vi "Teleop.vi"(10 "Match Info":T1={"Autonomous Elapsed Seconds"=0.0, "TeleOp Elapsed Seconds"=0.0, "Disabled Elapsed Seconds"=0.0, "Visited Autonomous"=FALSE, "Visited TeleOp"=FALSE, "Visited Disabled"=FALSE, "Autonomous Settings"={"Autonomous Style"=enum."Independent", "VI Refnum"=refnum}}, 11 "Call Context":T2) -> ()   [LabVIEW 2019]
doc: "This VI is called for each TeleOp packet received from the DS where the robot is not disabled. It is often used to read from the joysticks and update I/O or to update setpoints for timed control loops. It should complete and return within 20 milliseconds or it may miss DS packets."
uses:
  <vilib>/Rock Robotics/WPI/DriverStation/WPI_DriverStationDerivedRobotMode.ctl
  <vilib>/Rock Robotics/WPI/DriverStation/WPI_DriverStationMatch Info.ctl
  <vilib>/Rock Robotics/WPI/Solenoid/WPI_SolenoidValue.ctl
  <vilib>/Rock Robotics/WPI/ThirdParty/Phoenix-LabVIEW/Motor Controller/Controls/CTRE_Phoenix_MotorControl_ControlMode.ctl
  <vilib>/Rock Robotics/WPI/Utilities/WPI_GetSetVariantRefNum.vi
  <vilib>/Rock Robotics/Network Tables/NT Write Boolean Array.vi
  <vilib>/Rock Robotics/Network Tables/NT Write Numeric Array.vi
  <vilib>/Rock Robotics/Network Tables/NT Read Boolean.vi
  <vilib>/Rock Robotics/Network Tables/NT Read Number.vi
  <vilib>/Rock Robotics/WPI/Solenoid/WPI_SolenoidSetEnum.vi
  <vilib>/addons/control/pid/pid.llb/PID (DBL).vi
  <vilib>/Rock Robotics/Network Tables/NT Write Number.vi
  <vilib>/addons/control/pid/NI_PID_pid.lvlib
panel:
  out "Sample Slider 0":dbl(slide) scale=0.0..5.0
  out "Sample Boolean 1":bool
  out "Sample Boolean 0":bool
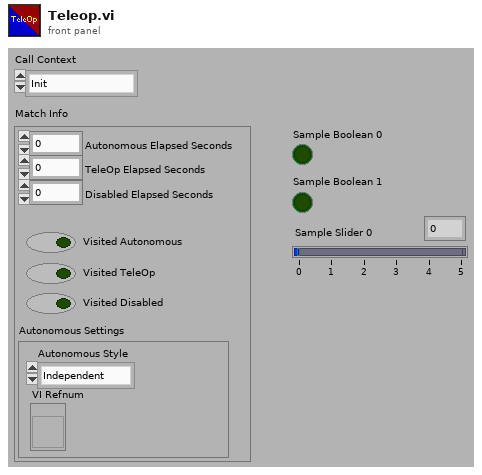
[diagram p1: front panel]
types:
  T1 = typedef "WPI_DriverStationMatch Info.ctl" = cluster{"Autonomous Elapsed Seconds":dbl, "TeleOp Elapsed Seconds":dbl, "Disabled Elapsed Seconds":dbl, "Visited Autonomous":bool, "Visited TeleOp":bool, "Visited Disabled":bool, "Autonomous Settings":cluster{"Autonomous Style":enum16{"Iterative", "Independent"}, "VI Refnum":refnum<vi>}}
  T2 = typedef "WPI_DriverStationDerivedRobotMode.ctl" = enum16{"Init", "Execute", "Stop"}
  T3 = typedef "CTRE_Phoenix_MotorControl_ControlMode.ctl" = u16
  T4 = typedef "WPI_SolenoidValue.ctl" = enum16{"Off", "On", "Forward", "Reverse"}
  T5 = typedef "WPI_RobotDriveDevRef.ctl" = cluster{"DevStatus":errorcluster, "Motors[]":T6[], "Square Inputs":bool, "Max Output":dbl}
  T6 = typedef "WPI_MotorControlDeviceRef.ctl" = cluster{"DeviceStatus":errorcluster, "Type":T7, "PWM":cluster{"PWM Channel":T8, "DeadBand":T9}, "CAN":cluster{"Device Number":u8, "SetOutput VI Ref":variant, "GetOutput VI Ref":variant, "Enable VI Ref":variant, "Disable VI Ref":variant, "Data":variant}, "Invert":bool, "DIO PWM":cluster{"PWM \"Enable\" Channel":T8, "DIOChannel":T10, "PWM Rate":dbl}}
  T7 = typedef "WPI_MotorControlType.ctl" = enum16{"PWM", "CAN", "DIO PWM"}
  T8 = typedef "FPGA_DIOPWMChannel.ctl" = enum8{"PWM 0", "PWM 1", "PWM 2", "PWM 3", "PWM 4", "PWM 5", "PWM 6", "PWM 7", "PWM 8", "PWM 9", "PWM MXP 0", "PWM MXP 1", "PWM MXP 2", "PWM MXP 3", "PWM MXP 4", "PWM MXP 5", "PWM MXP 6", "PWM MXP 7", "PWM MXP 8", "PWM MXP 9", "Invalid"}
  T9 = typedef "WPI_PWMDeadband.ctl" = cluster{"Name":string, "maxPositivePwm":i32, "minPositivePwm":i32, "centerPwm":i32, "maxNegativePwm":i32, "minNegativePwm":i32, "angularRange":u16}
  T10 = typedef "FPGA_DIOChannel.ctl" = enum8{"DIO 0", "DIO 1", "DIO 2", "DIO 3", "DIO 4", "DIO 5", "DIO 6", "DIO 7", "DIO 8", "DIO 9", "DIO MXP 0", "DIO MXP 1", "DIO MXP 2", "DIO MXP 3", "DIO MXP 4", "DIO MXP 5", "DIO MXP 6", "DIO MXP 7", "DIO MXP 8", "DIO MXP 9", "DIO MXP 10", "DIO MXP 11", "DIO MXP 12", "DIO MXP 13", "DIO MXP 14", "DIO MXP 15", "SPI Port CS1", "SPI Port CS2", "SPI Port CS3", "SPI Port MISO", "SPI Port MOSI", "Invalid"}
  T11 = typedef "WPI_JoystickDevRef.ctl" = cluster{"Device":T12}
  T12 = typedef "WPI_JoystickDeviceEnum.ctl" = enum16{"USB 0", "USB 1", "USB 2", "USB 3", "USB 4", "USB 5"}
  T13 = cluster{"Buttons[0]":bool, "Buttons[1]":bool, "Buttons[2]":bool, "Buttons[3]":bool, "Buttons[4]":bool, "Buttons[5]":bool, "Buttons[6]":bool, "Buttons[7]":bool, "Buttons[8]":bool}
  T14 = typedef "WPI_SolenoidDevRef.ctl" = cluster{"DevStatus":errorcluster, "Pneumatics Control Module":u8, "Forward Solenoid Channel":T15, "Reverse Solenoid Channel":T15}
  T15 = typedef "WPI_SolenoidChannel.ctl" = enum8{"Solenoid 0", "Solenoid 1", "Solenoid 2", "Solenoid 3", "Solenoid 4", "Solenoid 5", "Solenoid 6", "Solenoid 7", "Invalid"}
  T16 = cluster{"proportional gain (Kc)":dbl, "integral time (Ti, min)":dbl, "derivative time (Td, min)":dbl}
  T17 = typedef "WPI_SwitchDevRef.ctl" = cluster{"DevStatus":errorcluster, "DIO Channel":T10, "CntIndex":T18, "Normally Closed":bool}
  T18 = typedef "FPGA_CounterCtrSystemIndex.ctl" = enum8{"Ctr 0", "Ctr 1", "Ctr 2", "Ctr 3", "Ctr 4", "Ctr 5", "Ctr 6", "Ctr 7", "Invalid"}
  T19 = typedef "WPI_DigitalInputDevRef.ctl" = cluster{"DevStatus":errorcluster, "DIO Channel":T10}
  T20 = typedef "WPI_EncoderDevRef.ctl" = cluster{"DevStatus":errorcluster, "EncoderIndex":T21, "CounterIndex":T18, "DistancePerCount":dbl, "Decoding Type":T22}
  T21 = typedef "FPGA_EncoderIdx.ctl" = enum8{"Enc 0", "Enc 1", "Enc 2", "Enc 3", "Enc 4", "Enc 5", "Enc 6", "Enc 7", "Invalid"}
  T22 = typedef "WPI_EncoderType.ctl" = enum16{"1x", "2x", "4x"}
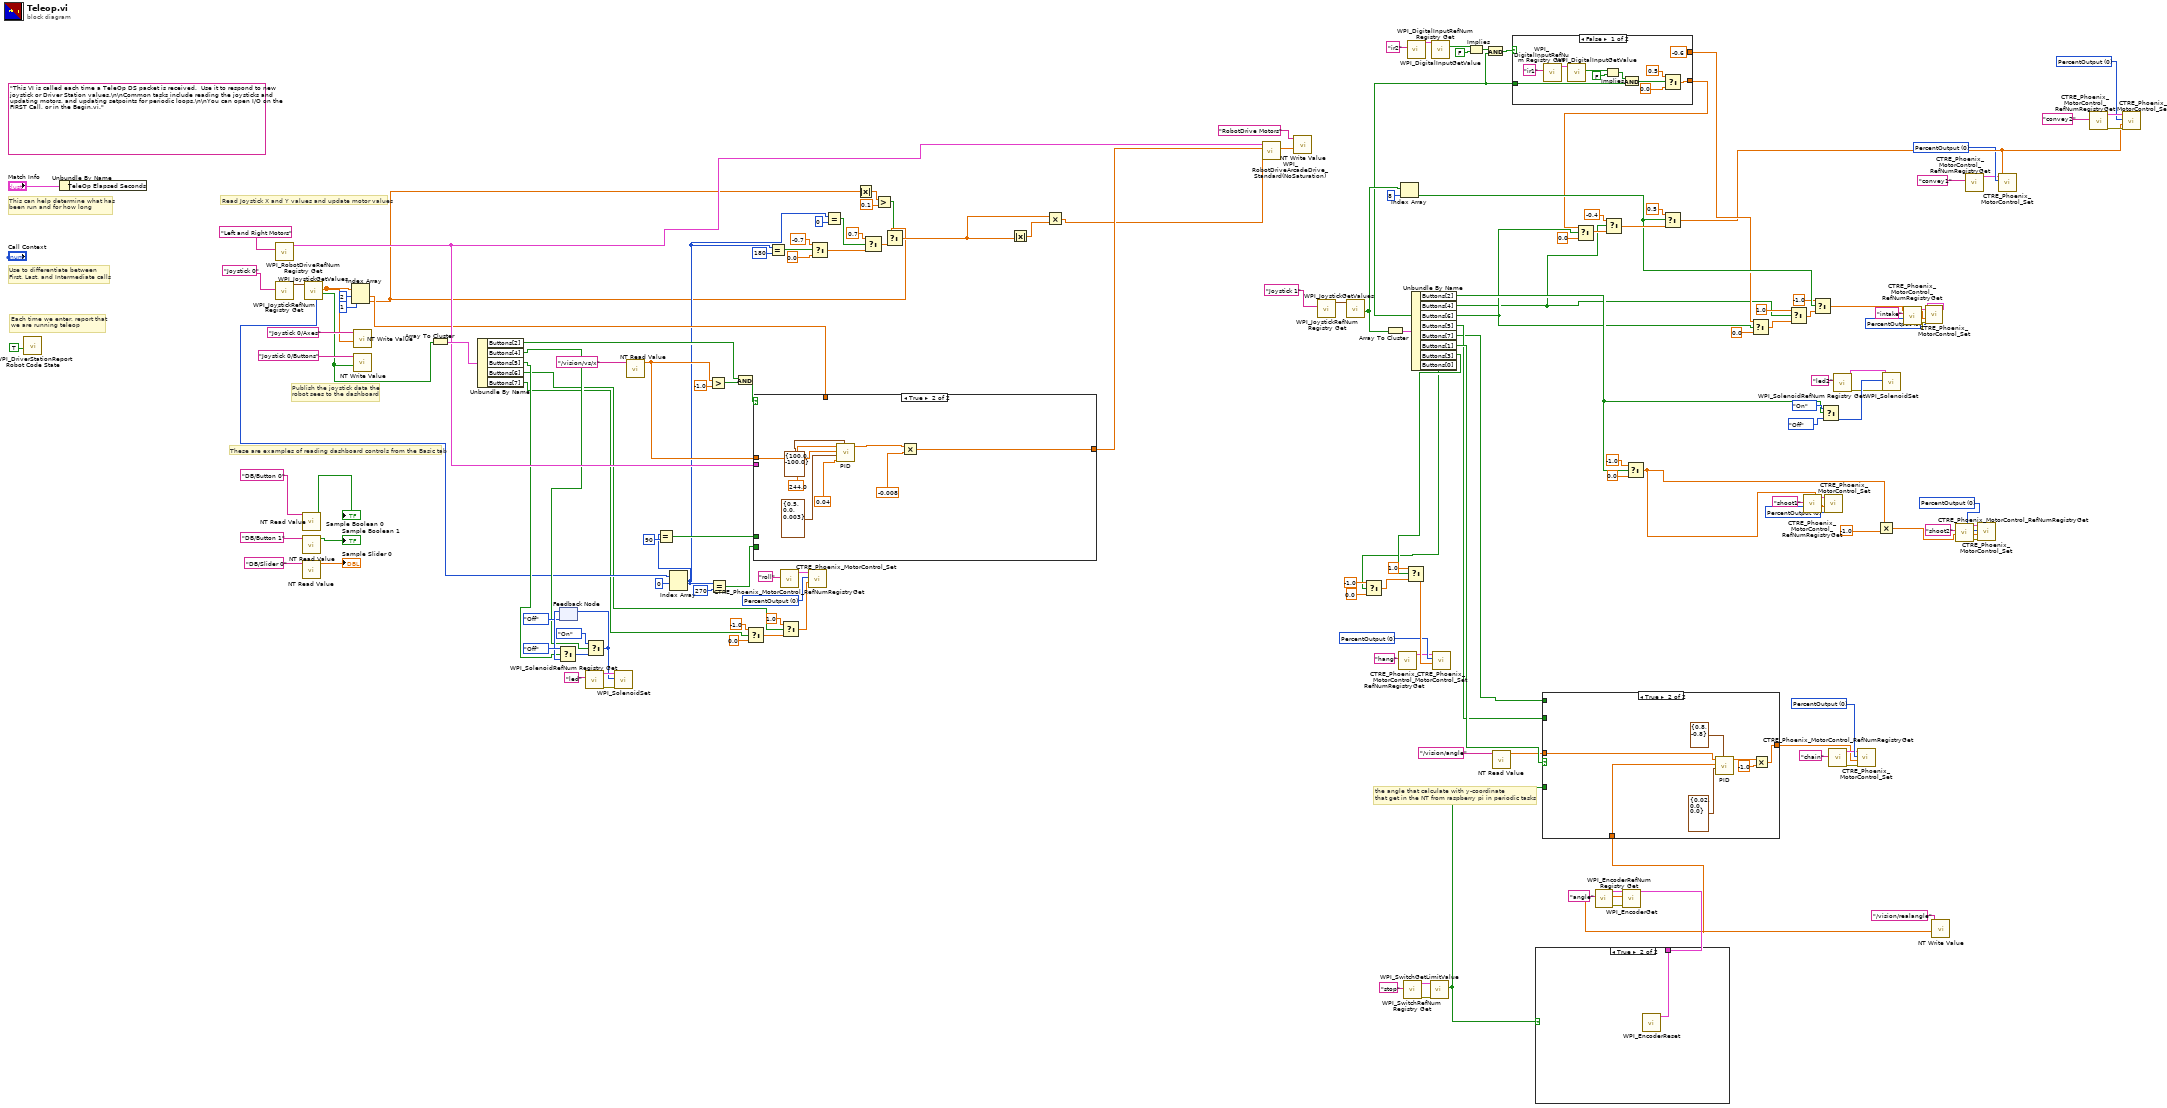
[diagram p0: block diagram]
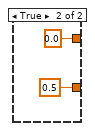
[diagram p2: hidden frame]
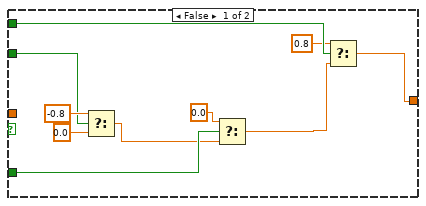
[diagram p3: hidden frame]
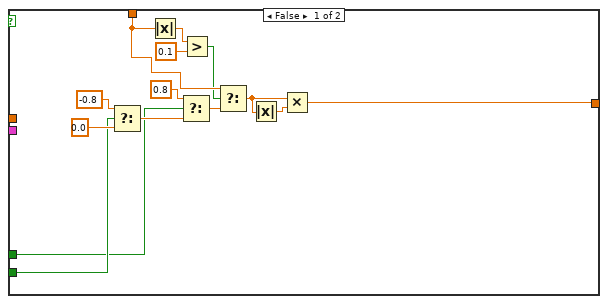
[diagram p5: hidden frame]
diagram:
  w4 = T3 0 items=["PercentOutput"=0, "Position"=1, "Velocity"=2, "Current"=3, "Follower"=5, "MotionProfile"=6, "MotionMagic"=7, "MotionProfileArc"=10, "Disabled"=15] ("Control Mode")
  w7 = T3 0 items=["PercentOutput"=0, "Position"=1, "Velocity"=2, "Current"=3, "Follower"=5, "MotionProfile"=6, "MotionMagic"=7, "MotionProfileArc"=10, "Disabled"=15] ("Control Mode")
  w34 = T3 0 items=["PercentOutput"=0, "Position"=1, "Velocity"=2, "Current"=3, "Follower"=5, "MotionProfile"=6, "MotionMagic"=7, "MotionProfileArc"=10, "Disabled"=15] ("Control Mode")
  w39 = T3 0 items=["PercentOutput"=0, "Position"=1, "Velocity"=2, "Current"=3, "Follower"=5, "MotionProfile"=6, "MotionMagic"=7, "MotionProfileArc"=10, "Disabled"=15] ("Control Mode")
  w85 = T3 0 items=["PercentOutput"=0, "Position"=1, "Velocity"=2, "Current"=3, "Follower"=5, "MotionProfile"=6, "MotionMagic"=7, "MotionProfileArc"=10, "Disabled"=15] ("Control Mode")
  w102 = T3 0 items=["PercentOutput"=0, "Position"=1, "Velocity"=2, "Current"=3, "Follower"=5, "MotionProfile"=6, "MotionMagic"=7, "MotionProfileArc"=10, "Disabled"=15] ("Control Mode")
  w114 = T3 0 items=["PercentOutput"=0, "Position"=1, "Velocity"=2, "Current"=3, "Follower"=5, "MotionProfile"=6, "MotionMagic"=7, "MotionProfileArc"=10, "Disabled"=15] ("Control Mode")
  w132 = T3 0 items=["PercentOutput"=0, "Position"=1, "Velocity"=2, "Current"=3, "Follower"=5, "MotionProfile"=6, "MotionMagic"=7, "MotionProfileArc"=10, "Disabled"=15] ("Control Mode")
  (unwired) "This VI is called each time a TeleOp DS packet is received.  Use it to respond to new joystick or Driver Station values.\n\nCommon tasks include reading the joysticks and updating motors, and updating setpoints for periodic loops.\n\nYou can open I/O on the FIRST Call, or in the Begin.vi."
  # "the angle that calculate with y-coordinate\nthat get in the NT from raspberry pi in periodic tasks"
  # "These are examples of reading dashboard controls from the Basic tab"
  # "Publish the joystick data the\nrobot sees to the dashboard"
  # "Each time we enter, report that\nwe are running teleop"
  # "Use to differentiate between\nFirst, Last, and Intermediate calls"
  # "This can help determine what has\nbeen run and for how long"
  # "Read Joystick X and Y values and update motor values"
  n1 = call <vilib>:"WPI_DriverStationReport Robot Code State.vi"("TeleOp"=TRUE ("Autonomous")) -> ()  [unwired: 10 in, 1 out]
  n2 = Unbundle By Name("Match Info") -> ()  [unwired: 1 out]
  n3 = call <vilib>:"WPI_RobotDriveRefNum Registry Get.vi"("refnum name"="Left and Right Motors") -> ("RobotDriveDevRef"=w143:T5)  [unwired: 1 in, 9 out]
  n4 = call <vilib>:"WPI_JoystickRefNum Registry Get.vi"("refnum name"="Joystick 0") -> ("JoystickDevRef"=w158:T11)  [unwired: 1 in, 9 out]
  n5 = call-poly <vilib>:"NT Read Value.vi"("Name"="DB/Button 0" ("refnum name")) -> ("Boolean"=→"Sample Boolean 0":bool)  [unwired: 9 in, 1 out]
  n6 = call-poly <vilib>:"NT Read Value.vi"("Name"="DB/Slider 0" ("refnum name")) -> ("Numeric"=→"Sample Slider 0":dbl)  [unwired: 9 in, 1 out]
  n7 = call-poly <vilib>:"NT Read Value.vi"("Name"="DB/Button 1" ("refnum name")) -> ("Boolean"=→"Sample Boolean 1":bool)  [unwired: 9 in, 1 out]
  n8 = call <vilib>:"WPI_JoystickGetValues.vi"("JoystickDevRef"=w158) -> ("Buttons"=w145:bool[], "Axes"=w154:dbl[], "POVs"=w79:i16[])  [unwired: 6 in, 2 out]
  n9 = Index Array(array=w154, index #1=2 ("index"), index #2=1 ("index")) -> (element #1=w94:dbl, element #2=w57:dbl)
  n10 = call-poly <vilib>:"NT Write Value.vi"("Numeric Array"=w154, "Name"="Joystick 0/Axes") -> ()  [unwired: 9 in, 1 out]
  n11 = call-poly <vilib>:"NT Write Value.vi"("Boolean Array"=w145, "Name"="Joystick 0/Buttons") -> ()  [unwired: 9 in, 1 out]
  n12 = Array To Cluster(array=w145) -> (cluster=w144:T13)
  n13 = Unbundle By Name(w144) -> ("Buttons[2]"=w96:bool, "Buttons[4]"=w116:bool, "Buttons[5]"=w115:bool, "Buttons[6]"=w72:bool, "Buttons[7]"=w71:bool)
  n14 = feedback #1(WPI_SolenoidValue."Off" ("Value")) -> (w119:T4)
  n15 = Select(t=WPI_SolenoidValue."Off" ("Value"), s=w115, f=w119) -> (s? t:f=w120:T4)
  n16 = call <vilib>:"WPI_SolenoidRefNum Registry Get.vi"("refnum name"="led") -> ("error out"=w125:errorcluster, "SolenoidDevRef"=w124:T14)  [unwired: 9 in]
  n17 = Select(t=WPI_SolenoidValue."On" ("Value"), s=w116, f=w120) -> (s? t:f=w117:T4)
  n18 = feedback-in #1(w117) -> ()
  n19 = call-poly <vilib>:"WPI_SolenoidSet.vi"("error in (no error)"=w125, "Value"=w117, "SolenoidDevRef"=w124) -> ()  [unwired: 7 in, 2 out]
  n20 = call-poly <vilib>:"NT Read Value.vi"("Name"="/vision/vs/x") -> ("Numeric"=w99:dbl)  [unwired: 9 in, 1 out]
  n21 = Index Array(array=w79, index #1=0 ("index")) -> (element #1=w61:i16)  [unwired: 1 in, 1 out]
  n22 = Equal?(x=w61, y=i16 90) -> (x = y?=w76:bool)
  n23 = Greater?(x=w99, y=-1.0) -> (0:w97:bool)
  n24 = Equal?(x=w61, y=i16 270) -> (x = y?=w77:bool)
  n25 = And(x=w96, y=w97) -> (x .and. y?=w95:bool)
  n26 = Select(t=-1.0, s=w71, f=0.0) -> (s? t:f=w82:dbl)
  n27 = case shown="True" w95 {
    tunnel: w143 -> [_ _]
    tunnel: w99 -> [_ w183]
    tunnel: [w162 w177] -> w93
    tunnel: w94 -> [w166 _]
    tunnel: w77 -> [w170 _]
    tunnel: w76 -> [w169 _]
    frame False {
      n28 = Select(t=-0.8, s=w170, f=0.0) -> (s? t:f=w174:dbl)
      n29 = Absolute Value(x=w166) -> (abs(x)=w165:dbl)
      n30 = Select(t=0.8, s=w169, f=w174) -> (s? t:f=w171:dbl)
      n31 = Greater?(x=w165, y=0.1) -> (0:w163:bool)
      n32 = Select(t=w166, s=w163, f=w171) -> (s? t:f=w167:dbl)
      n33 = Absolute Value(x=w167) -> (abs(x)=w168:dbl)
      n34 = Multiply(x=w167, y=w168) -> (x*y=w162:dbl)
    }
    frame True {
      n35 = call-poly <vilib>:"PID.vi"("output range"=cluster{"output high":dbl, "output low":dbl} {"output high"=100.0, "output low"=-100.0}, "dt (s)"=0.04, "PID gains"=T16 {"proportional gain (Kc)"=0.5, "integral time (Ti, min)"=0.0, "derivative time (Td, min)"=0.003}, "process variable"=w183, "setpoint"=244.0) -> ("output"=w179:dbl)  [unwired: 5 in, 1 out]
      n36 = Multiply(x=w179, y=-0.008) -> (x*y=w177:dbl)
    }
  }
  n37 = Equal?(x=w61, y=i16 180) -> (x = y?=w62:bool)
  n38 = call <vilib>:"CTRE_Phoenix_MotorControl_RefNumRegistryGet.vi"("refnum name"="roll") -> ("PhoenixMotorControlDevRef"=w87:T6)  [unwired: 9 in, 1 out]
  n39 = Select(t=1.0, s=w72, f=w82) -> (s? t:f=w78:dbl)
  n40 = call <vilib>:"CTRE_Phoenix_MotorControl_Set.vi"("Output"=w78, "Control Mode"=w85, "PhoenixMotorControlDevRef"=w87) -> ()  [unwired: 7 in, 2 out]
  n41 = Select(t=-0.7, s=w62, f=0.0) -> (s? t:f=w67:dbl)
  n42 = Equal?(x=w61, y=i16 0) -> (x = y?=w63:bool)
  n43 = Absolute Value(x=w57) -> (abs(x)=w56:dbl)
  n44 = Select(t=0.7, s=w63, f=w67) -> (s? t:f=w70:dbl)
  n45 = Greater?(x=w56, y=0.1) -> (0:w54:bool)
  n46 = Select(t=w57, s=w54, f=w70) -> (s? t:f=w59:dbl)
  n47 = Absolute Value(x=w59) -> (abs(x)=w60:dbl)
  n48 = Multiply(x=w59, y=w60) -> (x*y=w58:dbl)
  n49 = call <vilib>:"WPI_RobotDriveArcadeDrive_Standard(NoSaturation).vi"("Y axis value"=w58, "X axis value"=w93, "RobotDriveDevRef"=w143) -> ("Motor Values"=w147:dbl[])  [unwired: 1 in, 7 out]
  n50 = call-poly <vilib>:"NT Write Value.vi"("Numeric Array"=w147, "Name"="RobotDrive Motors") -> ()  [unwired: 9 in, 1 out]
  n51 = call <vilib>:"WPI_JoystickRefNum Registry Get.vi"("refnum name"="Joystick 1") -> ("JoystickDevRef"=w139:T11)  [unwired: 1 in, 9 out]
  n52 = call <vilib>:"WPI_JoystickGetValues.vi"("JoystickDevRef"=w139) -> ("Buttons"=w47:bool[])  [unwired: 6 in, 4 out]
  n53 = Array To Cluster(array=w47) -> (cluster=w137:T13)
  n54 = call <vilib>:"CTRE_Phoenix_MotorControl_RefNumRegistryGet.vi"("refnum name"="hang") -> ("PhoenixMotorControlDevRef"=w100:T6)  [unwired: 9 in, 1 out]
  n55 = Index Array(array=w47, index=8) -> (element=w44:bool)
  n56 = call <vilib>:"WPI_SwitchRefNum Registry Get.vi"("refnum name"="stop") -> ("error out"=w90:errorcluster, "SwitchDevRef"=w89:T17)  [unwired: 9 in]
  n57 = call <vilib>:"WPI_DigitalInputRefNum Registry Get.vi"("refnum name"="ir2") -> ("DigitalInputDevRef"=w20:T19)  [unwired: 9 in, 1 out]
  n58 = Unbundle By Name(w137) -> ("Buttons[2]"=w48:bool, "Buttons[4]"=w1:bool, "Buttons[6]"=w2:bool, "Buttons[5]"=w28:bool, "Buttons[7]"=w27:bool, "Buttons[1]"=w29:bool, "Buttons[3]"=w73:bool, "Buttons[0]"=w53:bool)
  n59 = Select(t=-1.0, s=w53, f=0.0) -> (s? t:f=w106:dbl)
  n60 = Select(t=1.0, s=w73, f=w106) -> (s? t:f=w103:dbl)
  n61 = call <vilib>:"WPI_SwitchGetLimitValue.vi"("error in (no error)"=w90, "SwitchDevRef"=w89) -> ("Switch Pressed"=w25:bool)  [unwired: 7 in, 2 out]
  n62 = call <vilib>:"WPI_DigitalInputGetValue.vi"("DigitalInputDevRef"=w20) -> ("Value"=w22:bool)  [unwired: 8 in, 2 out]
  n63 = call <vilib>:"CTRE_Phoenix_MotorControl_Set.vi"("Output"=w103, "Control Mode"=w102, "PhoenixMotorControlDevRef"=w100) -> ()  [unwired: 7 in, 2 out]
  n64 = Implies(1:FALSE ("y"), 2:w22) -> (0:w18:bool)
  n65 = And(x=w18, y=w2) -> (x .and. y?=w19:bool)
  n66 = call-poly <vilib>:"NT Read Value.vi"("Name"="/vision/angle") -> ("Numeric"=w26:dbl)  [unwired: 9 in, 1 out]
  n67 = case shown="False" w19 {
    tunnel: [-0.6 0.0] -> w15
    tunnel: [w185 0.5] -> w11
    tunnel: w2 -> [w188 _]
    frame False {
      n68 = call <vilib>:"WPI_DigitalInputRefNum Registry Get.vi"("refnum name"="ir1") -> ("DigitalInputDevRef"=w193:T19)  [unwired: 9 in, 1 out]
      n69 = call <vilib>:"WPI_DigitalInputGetValue.vi"("DigitalInputDevRef"=w193) -> ("Value"=w192:bool)  [unwired: 8 in, 2 out]
      n70 = Implies(1:FALSE ("y"), 2:w192) -> (0:w191:bool)
      n71 = And(x=w191, y=w188) -> (x .and. y?=w187:bool)
      n72 = Select(t=0.5, s=w187, f=0.0) -> (s? t:f=w185:dbl)
    }
    frame True {
    }
  }
  n73 = Select(t=w11, s=w2, f=0.0) -> (s? t:f=w13:dbl)
  n74 = call <vilib>:"WPI_EncoderRefNum Registry Get.vi"("refnum name"="angle") -> ("error out"=w109:errorcluster, "EncoderDevRef"=w110:T20)  [unwired: 9 in]
  n75 = Select(t=-0.4, s=w1, f=w13) -> (s? t:f=w50:dbl)
  n76 = call <vilib>:"WPI_EncoderGet.vi"("error in (no error)"=w109, "EncoderDevRef"=w110) -> ("Distance"=w30:dbl, "EncoderDevRef"=w92:T20)  [unwired: 4 in, 4 out]
  n77 = case shown="True" w25 {
    tunnel: w92 -> [_ w197]
    frame False {
    }
    frame True {
      n78 = call <vilib>:"WPI_EncoderReset.vi"("EncoderDevRef"=w197) -> ()  [unwired: 9 in, 2 out]
    }
  }
  n79 = case shown="True" w29 {
    tunnel: w30 -> [_ w210]
    tunnel: w28 -> [w202 _]
    tunnel: w27 -> [w207 _]
    tunnel: w26 -> [_ w209]
    tunnel: w25 -> [w203 _]
    tunnel: [w201 w208] -> w24
    frame False {
      n80 = Select(t=-0.8, s=w202, f=0.0) -> (s? t:f=w200:dbl)
      n81 = Select(t=0.0, s=w203, f=w200) -> (s? t:f=w198:dbl)
      n82 = Select(t=0.8, s=w207, f=w198) -> (s? t:f=w201:dbl)
    }
    frame True {
      n83 = call-poly <vilib>:"PID.vi"("output range"=cluster{"output high":dbl, "output low":dbl} {"output high"=0.8, "output low"=-0.8}, "PID gains"=T16 {"proportional gain (Kc)"=0.02, "integral time (Ti, min)"=0.0, "derivative time (Td, min)"=0.0}, "process variable"=w210, "setpoint"=w209) -> ("output"=w213:dbl)  [unwired: 6 in, 1 out]
      n84 = Multiply(x=w213, y=-1.0) -> (x*y=w208:dbl)
    }
  }
  n85 = Select(t=-1.0, s=w48, f=0.0) -> (s? t:f=w31:dbl)
  n86 = Select(t=0.5, s=w44, f=w50) -> (s? t:f=w6:dbl)
  n87 = Select(t=w15, s=w2, f=0.0) -> (s? t:f=w17:dbl)
  n88 = Select(t=1.0, s=w1, f=w17) -> (s? t:f=w45:dbl)
  n89 = call <vilib>:"CTRE_Phoenix_MotorControl_RefNumRegistryGet.vi"("refnum name"="shoot1") -> ("PhoenixMotorControlDevRef"=w32:T6)  [unwired: 9 in, 1 out]
  n90 = Select(t=-1.0, s=w44, f=w45) -> (s? t:f=w42:dbl)
  n91 = Select(t=WPI_SolenoidValue."On" ("Value"), s=w48, f=WPI_SolenoidValue."Off") -> (s? t:f=w131:T4)
  n92 = call <vilib>:"CTRE_Phoenix_MotorControl_Set.vi"("Output"=w31, "Control Mode"=w34, "PhoenixMotorControlDevRef"=w32) -> ()  [unwired: 7 in, 2 out]
  n93 = call <vilib>:"CTRE_Phoenix_MotorControl_RefNumRegistryGet.vi"("refnum name"="chain") -> ("error out"=w111:errorcluster, "PhoenixMotorControlDevRef"=w112:T6)  [unwired: 9 in]
  n94 = call <vilib>:"WPI_SolenoidRefNum Registry Get.vi"("refnum name"="led2") -> ("error out"=w128:errorcluster, "SolenoidDevRef"=w129:T14)  [unwired: 9 in]
  n95 = call <vilib>:"CTRE_Phoenix_MotorControl_Set.vi"("error in (no error)"=w111, "Output"=w24, "Control Mode"=w114, "PhoenixMotorControlDevRef"=w112) -> ()  [unwired: 6 in, 2 out]
  n96 = Multiply(x=w31, y=-1.0) -> (x*y=w40:dbl)
  n97 = call-poly <vilib>:"WPI_SolenoidSet.vi"("error in (no error)"=w128, "Value"=w131, "SolenoidDevRef"=w129) -> ()  [unwired: 7 in, 2 out]
  n98 = call <vilib>:"CTRE_Phoenix_MotorControl_RefNumRegistryGet.vi"("refnum name"="intake") -> ("error out"=w136:errorcluster, "PhoenixMotorControlDevRef"=w135:T6)  [unwired: 9 in]
  n99 = call <vilib>:"CTRE_Phoenix_MotorControl_Set.vi"("error in (no error)"=w136, "Output"=w42, "Control Mode"=w132, "PhoenixMotorControlDevRef"=w135) -> ()  [unwired: 6 in, 2 out]
  n100 = call-poly <vilib>:"NT Write Value.vi"("Numeric"=w30, "Name"="/vision/realangle") -> ()  [unwired: 9 in, 1 out]
  n101 = call <vilib>:"CTRE_Phoenix_MotorControl_RefNumRegistryGet.vi"("refnum name"="shoot2") -> ("error out"=w37:errorcluster, "PhoenixMotorControlDevRef"=w38:T6)  [unwired: 9 in]
  n102 = call <vilib>:"CTRE_Phoenix_MotorControl_RefNumRegistryGet.vi"("refnum name"="convey1") -> ("PhoenixMotorControlDevRef"=w3:T6)  [unwired: 9 in, 1 out]
  n103 = call <vilib>:"CTRE_Phoenix_MotorControl_Set.vi"("error in (no error)"=w37, "Output"=w40, "Control Mode"=w39, "PhoenixMotorControlDevRef"=w38) -> ()  [unwired: 6 in, 2 out]
  n104 = call <vilib>:"CTRE_Phoenix_MotorControl_Set.vi"("Output"=w6, "Control Mode"=w4, "PhoenixMotorControlDevRef"=w3) -> ()  [unwired: 7 in, 2 out]
  n105 = call <vilib>:"CTRE_Phoenix_MotorControl_RefNumRegistryGet.vi"("refnum name"="convey2") -> ("error out"=w10:errorcluster, "PhoenixMotorControlDevRef"=w9:T6)  [unwired: 9 in]
  n106 = call <vilib>:"CTRE_Phoenix_MotorControl_Set.vi"("error in (no error)"=w10, "Output"=w6, "Control Mode"=w7, "PhoenixMotorControlDevRef"=w9) -> ()  [unwired: 6 in, 2 out]
